vi "Add To Display.vi"(8 "error in (no error)":errorcluster, 9 "Decimal Count In":u8, 10 "Display In":ext, 11 "Number In":dbl) -> (0 "error out":errorcluster, 1 "Decimal Count Out":u8, 2 "Display Out":ext)   [LabVIEW 2014]
doc: "This VI applies a decimal and increments the decimal count if we are in decimal mode (decimal count > 0).\n\nAuthor: Erik Johnson, National Instruments"
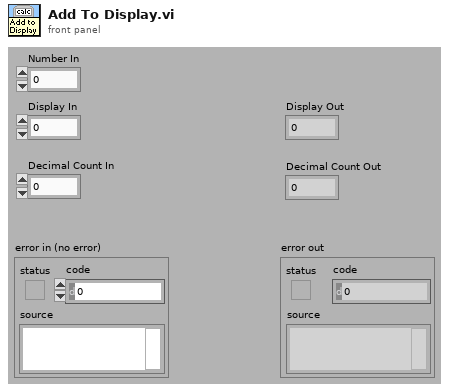
[diagram p1: front panel]
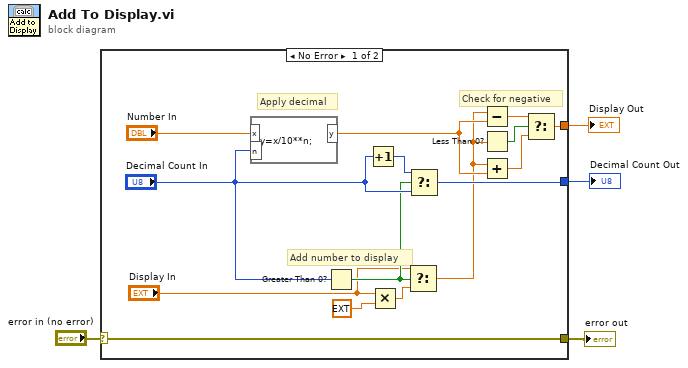
[diagram p0: block diagram]
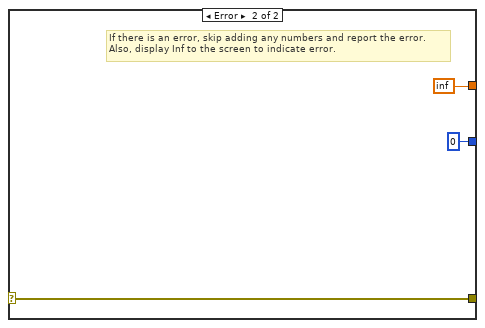
[diagram p2: hidden frame]
diagram:
  n1 = case shown="No Error" "error in (no error)" {
    selector: "error in (no error)" -> [w5 w22]
    tunnel: [w19 u8 0 ("Decimal Count In")] -> w4
    tunnel: [w7 inf] -> w3
    tunnel: [w5 w22] -> w1
    frame No Error {
      # "Add number to display"
      # "Check for negative"
      # "Apply decimal"
      n2 = formula code="y=x/10**n;"("x"="Number In", "n"="Decimal Count In") -> ("y"=w9:dbl)
      n3 = Greater Than 0?(x="Decimal Count In") -> (x > 0?=w13:bool)
      n4 = Increment(x="Decimal Count In") -> (x+1=w15:u8)
      n5 = Multiply(x="Display In", y=ext 10.0) -> (x*y=w17:ext)
      n6 = Select(t="Display In", s=w13, f=w17) -> (s? t:f=w8:ext)
      n7 = Select(t=w15, s=w13, f="Decimal Count In") -> (s? t:f=w19:u8)
      n8 = Subtract(x=w8, y=w9) -> (x-y=w12:ext)
      n9 = Less Than 0?(x=w8) -> (x < 0?=w10:bool)
      n10 = Add(x=w8, y=w9) -> (x+y=w11:ext)
      n11 = Select(t=w12, s=w10, f=w11) -> (s? t:f=w7:ext)
    }
    frame Error {
      # "If there is an error, skip adding any numbers and report the error.\nAlso, display Inf to the screen to indicate error."
    }
  }
  "Display Out" <- w3
  "Decimal Count Out" <- w4
  "error out" <- w1
